vi "OutputToXML.vi"(8 "error in (no error)":errorcluster, 11 "AppPluginsBase in":refnum<class "AppPluginsBase.lvclass">) -> (0 "error out":errorcluster, 2 "AppOutputData out":variant)   [LabVIEW 2014, in "AppPlugins.lvlib" / "AppPluginsBase.lvclass"]
uses:
  AppPluginsBase.lvclass
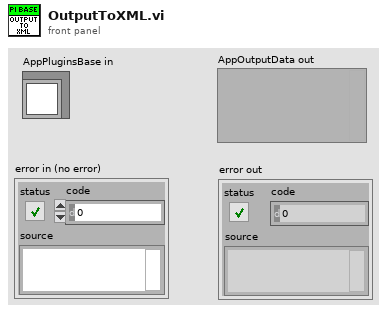
[diagram p1: front panel]
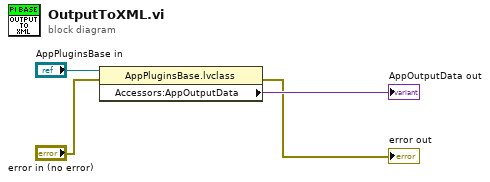
[diagram p0: block diagram]
diagram:
  n1 = property class="AppPluginsBase.lvclass"(reference="AppPluginsBase in", error in="error in (no error)") -> (error out=→"error out":errorcluster, "Accessors:AppOutputData"=→"AppOutputData out":variant)  [unwired: 1 out]
